vi "Midi In.vi"(8 "error in":errorcluster, 10 "Queue Name":string="Midi In", 11 "Midi Controller Name":refnum<visa-resource-name>) -> (0 "error out":errorcluster)   [LabVIEW 2014]
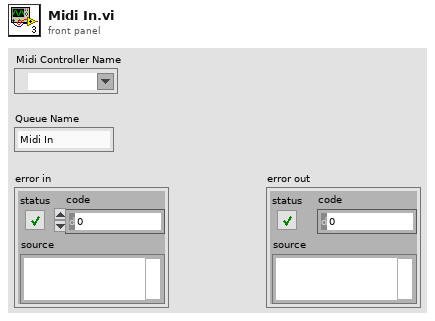
[diagram p1: front panel]
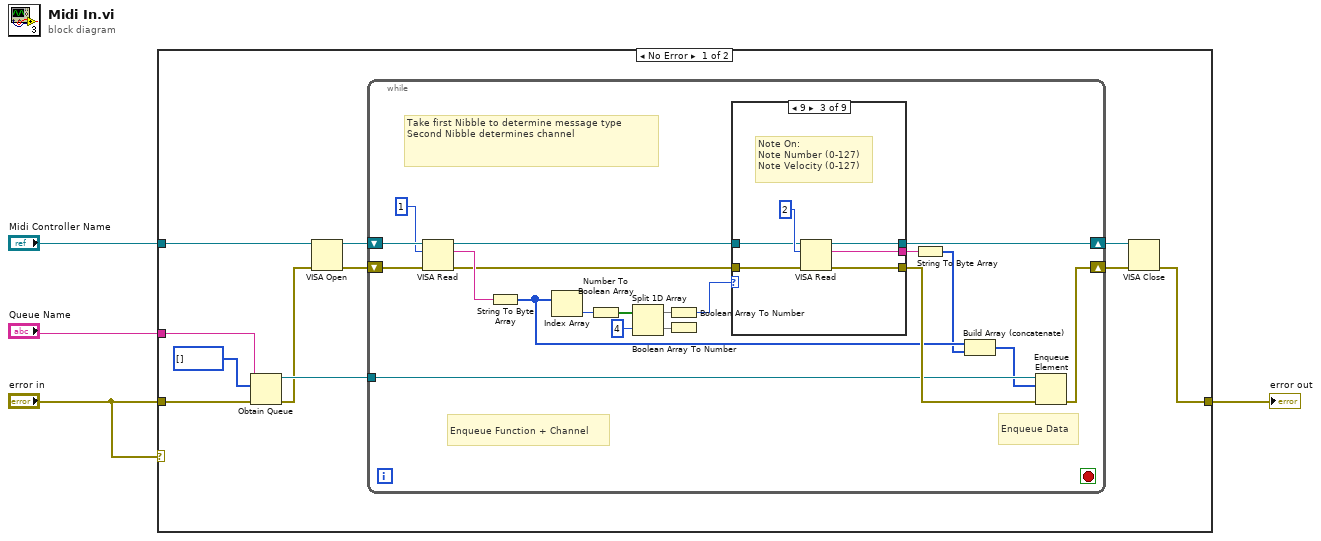
[diagram p0: block diagram]
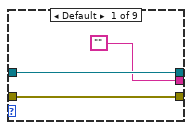
[diagram p2: hidden frame]
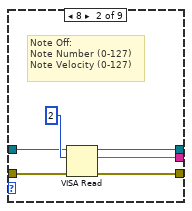
[diagram p3: hidden frame]
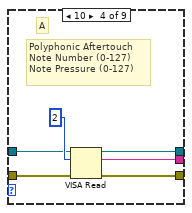
[diagram p4: hidden frame]
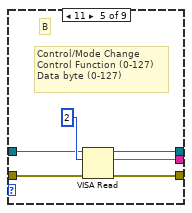
[diagram p5: hidden frame]
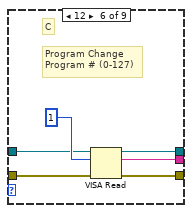
[diagram p6: hidden frame]
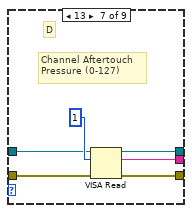
[diagram p7: hidden frame]
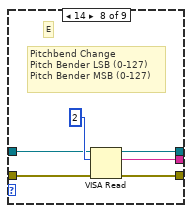
[diagram p8: hidden frame]
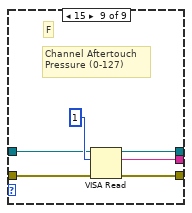
[diagram p9: hidden frame]
diagram:
  n1 = case shown="No Error" "error in" {
    tunnel: "error in" -> [w11 w87]
    tunnel: [w5 w87] -> w1
    tunnel: "Queue Name" -> [w10 _]
    tunnel: "Midi Controller Name" -> [w9 _]
    frame No Error {
      n2 = Obtain Queue(name (unnamed)=w10, element data type=u8[] [] ("unsigned byte array"), error in (no error)=w11) -> (queue out=w13:refnum<queue>, error out=w12:errorcluster)  [unwired: 2 in, 1 out]
      n3 = VISA Open(error in (no error)=w12, VISA resource name=w9) -> (VISA resource name=w15:refnum<visa-resource-name>, error out=w14:errorcluster)  [unwired: 3 in]
      n4 = while {
        shift-right: [w32] -> w7
        shift-left: w15 -> [w35]
        tunnel: w13 -> [w22]
        shift-right: [w23] -> w6
        shift-left: w14 -> [w31]
        stop <- _ stop-if-true
        # "Enqueue Data"
        # "Enqueue Function + Channel"
        # "Take first Nibble to determine message type\nSecond Nibble determines channel"
        n5 = VISA Read(VISA resource name=w35, byte count=u32 1, error in (no error)=w31) -> (VISA resource name out=w33:refnum<visa-resource-name>, read buffer=w30:string, error out=w21:errorcluster)  [unwired: 1 out]
        n6 = String To Byte Array(string=w30) -> (unsigned byte array=w19:u8[])
        n7 = Index Array(array=w19) -> (element=w29:u8)  [unwired: 1 in]
        n8 = Number To Boolean Array(number=w29) -> (Boolean array=w28:bool[])
        n9 = Split 1D Array(array=w28, index=4) -> (first subarray=w26:bool[], second subarray=w16:bool[])
        n10 = Boolean Array To Number(Boolean array=w26) -> (number=w25:u32)
        n11 = Boolean Array To Number(Boolean array=w16) -> ()  [unwired: 1 out]
        n12 = case shown="9" w25 {
          tunnel: w33 -> [w38 w43 w49 w55 w61 w67 w73 w79 w85]
          tunnel: [w38 w42 w48 w54 w60 w66 w72 w78 w84] -> w32
          tunnel: ["" w41 w47 w52 w59 w64 w70 w76 w82] -> w20
          tunnel: [w36 w40 w46 w53 w58 w65 w71 w77 w83] -> w24
          tunnel: w21 -> [w36 w39 w45 w51 w57 w63 w69 w75 w81]
          frame Default {
          }
          frame 8 {
            # "Note Off: \nNote Number (0-127)\nNote Velocity (0-127)"
            n13 = VISA Read(VISA resource name=w43, byte count=u32 2, error in (no error)=w39) -> (VISA resource name out=w42:refnum<visa-resource-name>, read buffer=w41:string, error out=w40:errorcluster)  [unwired: 1 out]
          }
          frame 9 {
            # "Note On: \nNote Number (0-127)\nNote Velocity (0-127)"
            n14 = VISA Read(VISA resource name=w49, byte count=u32 2, error in (no error)=w45) -> (VISA resource name out=w48:refnum<visa-resource-name>, read buffer=w47:string, error out=w46:errorcluster)  [unwired: 1 out]
          }
          frame 10 {
            # "A"
            # "Polyphonic Aftertouch\nNote Number (0-127)\nNote Pressure (0-127)"
            n15 = VISA Read(VISA resource name=w55, byte count=u32 2, error in (no error)=w51) -> (VISA resource name out=w54:refnum<visa-resource-name>, read buffer=w52:string, error out=w53:errorcluster)  [unwired: 1 out]
          }
          frame 11 {
            # "B"
            # "Control/Mode Change\nControl Function (0-127)\nData byte (0-127)"
            n16 = VISA Read(VISA resource name=w61, byte count=u32 2, error in (no error)=w57) -> (VISA resource name out=w60:refnum<visa-resource-name>, read buffer=w59:string, error out=w58:errorcluster)  [unwired: 1 out]
          }
          frame 12 {
            # "C"
            # "Program Change\nProgram # (0-127)"
            n17 = VISA Read(VISA resource name=w67, byte count=u32 1, error in (no error)=w63) -> (VISA resource name out=w66:refnum<visa-resource-name>, read buffer=w64:string, error out=w65:errorcluster)  [unwired: 1 out]
          }
          frame 13 {
            # "Channel Aftertouch\nPressure (0-127)"
            # "D"
            n18 = VISA Read(VISA resource name=w73, byte count=u32 1, error in (no error)=w69) -> (VISA resource name out=w72:refnum<visa-resource-name>, read buffer=w70:string, error out=w71:errorcluster)  [unwired: 1 out]
          }
          frame 14 {
            # "E"
            # "Pitchbend Change\nPitch Bender LSB (0-127)\nPitch Bender MSB (0-127)"
            n19 = VISA Read(VISA resource name=w79, byte count=u32 2, error in (no error)=w75) -> (VISA resource name out=w78:refnum<visa-resource-name>, read buffer=w76:string, error out=w77:errorcluster)  [unwired: 1 out]
          }
          frame 15 {
            # "F"
            # "Channel Aftertouch\nPressure (0-127)"
            n20 = VISA Read(VISA resource name=w85, byte count=u32 1, error in (no error)=w81) -> (VISA resource name out=w84:refnum<visa-resource-name>, read buffer=w82:string, error out=w83:errorcluster)  [unwired: 1 out]
          }
        }
        n21 = String To Byte Array(string=w20) -> (unsigned byte array=w18:u8[])
        n22 = Build Array (concatenate)(w19, w18) -> (w17:u8[])
        n23 = Enqueue Element(queue=w22, element=w17, error in (no error)=w24) -> (error out=w23:errorcluster)  [unwired: 1 in, 2 out]
      }
      n24 = VISA Close(VISA resource name=w7, error in (no error)=w6) -> (error out=w5:errorcluster)
    }
    frame Error {
    }
  }
  "error out" <- w1
